vi "Obtain New DAQ Data Notifier.vi"(1 "Notifier Name":string) -> (0 "DAQ Data Notifier":refnum<notifier>)   [LabVIEW 2013]
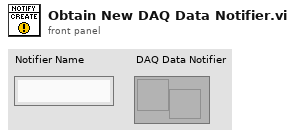
[diagram p1: front panel]
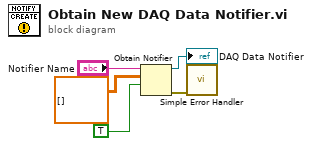
[diagram p0: block diagram]
diagram:
  n1 = Obtain Notifier(name (unnamed)="Notifier Name", notification data type=dbl[][] [] ("Data"), create if not found? (T)=TRUE) -> (notifier out=→"DAQ Data Notifier":refnum<notifier>, error out=w1:errorcluster)  [unwired: 1 in, 1 out]
  n2 = call <vilib>:"Simple Error Handler.vi"("error in (no error)"=w1) -> ()  [unwired: 4 in, 5 out]
